vi "Read On-the-fly.vi"(8 "error in (no error)":errorcluster, 11 "ResultProcessor Config in":refnum<class "ResultProcessor Config.lvclass">) -> (0 "error out":errorcluster, 2 "On-the-fly?":bool, 3 "ResultProcessor Config out":refnum<class "ResultProcessor Config.lvclass">)   [LabVIEW 2015, in "ResultProcessor Config.lvclass"]
uses:
  ResultProcessor Config.lvclass
  ResultProcessor Config.lvclass/ResultProcessor Config.ctl
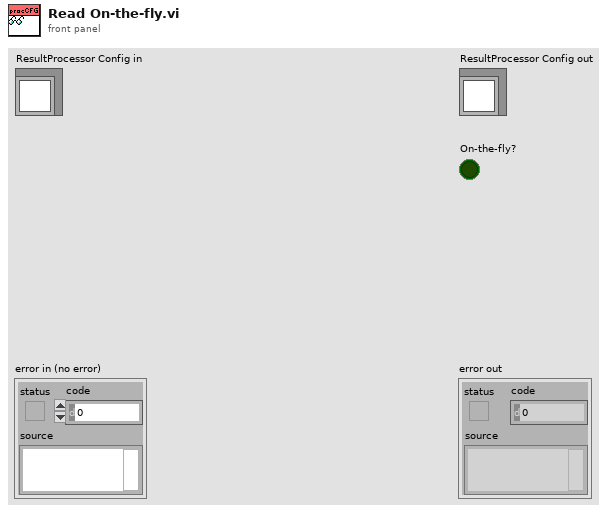
[diagram p1: front panel]
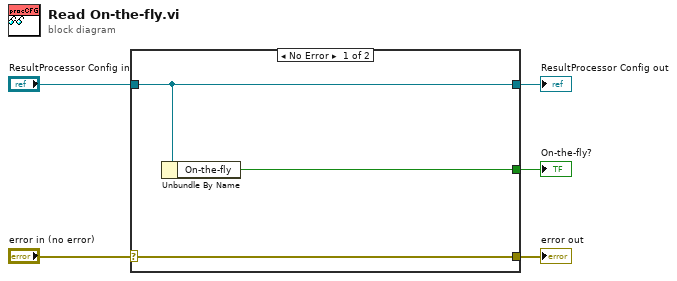
[diagram p0: block diagram]
diagram:
  n1 = case shown="No Error" "error in (no error)" {
    selector: "error in (no error)" -> [w8 w9]
    tunnel: [w8 w9] -> w4
    tunnel: [w7 w10] -> w2
    tunnel: "ResultProcessor Config in" -> [w7 w10]
    tunnel: [w6 _] -> w1
    frame No Error {
      n2 = Unbundle By Name(w7) -> ("On-the-fly"=w6:bool)
    }
    frame Error {
    }
  }
  "error out" <- w4
  "ResultProcessor Config out" <- w2
  "On-the-fly?" <- w1
